vi "bats.parser.test.vi"() -> ()   [LabVIEW 2020]
uses:
  <vilib>/Platform/TimedLoop/XDataNode/XDataNode.xnode
  <vilib>/Platform/TimedLoop/XDataNode/nitl_modes.ctl
  <vilib>/Platform/TimedLoop/XDataNode/XDNodeRunTimeDep.lvlib
  <vilib>/Platform/TimedLoop/XDataNode/wakeup.ctl
  <vilib>/Platform/TimedLoop/XDataNode/timing_clust.ctl
  <vilib>/rvi/LocalResourceManager/LocalResourceManager.xnode
  <vilib>/rvi/DataTransferAndStorage/Container/XNode/niFpgaContainer.xnode
  <vilib>/rvi/FIFO/Fifo_Resource/niFpgaFifoEmulationRefIn.vi
  <vilib>/rvi/interface/RandomDataEmulation/nirviRandomDataFpgaMultiElementTemplate.vi
  <vilib>/rvi/FIFO/Fifo_Resource/nirvififoEmulationRead.vi
  Market.Data.Common/fpga/fpganow.common.fpga.lvlib
  <instrlib>/_niInstr/Network/IPv4/UDP/Data Stream/v1/niInstr IPv4 UDP Data Stream v1.lvclass
  <instrlib>/_niInstr/Network/IPv4/UDP/Data Stream/v1/Write Data Stream.vi
  <vilib>/rvi/DataTransferAndStorage/Container/Common/niFpgaContainerGetUniqueNameForEmu.vi
  <vilib>/rvi/DataTransferAndStorage/Container/Common/niFpgaContainerSetEmuInfo.vi
  <vilib>/rvi/eio/common/nirviEmuReportErrorAndStop.vi
  <instrlib>/_niInstr/Network/Ethernet/Utility/v1/FPGA/Network Data Stream.ctl
  <instrlib>/_niInstr/Network/Ethernet/Utility/v1/FPGA/niInstr Ethernet Utilities FPGA v1.lvlib
panel:
  out "byte":u8[](array[numeric]) format="%.0x"
  out "enabled":bool[](array[boolean])
  in  "Data Stream":T1={"data"=[0, 0, 0, 0, 0, 0, 0, 0], "data valid"=FALSE, "byte enables"=[FALSE, FALSE, FALSE, FALSE, FALSE, FALSE, FALSE, FALSE]}
  in  "niInstr IPv4 UDP Data Stream out":refnum<class "niInstr IPv4 UDP Data Stream v1.lvclass">
  out "Element":u64[](array[numeric])
  in  "reset":bool
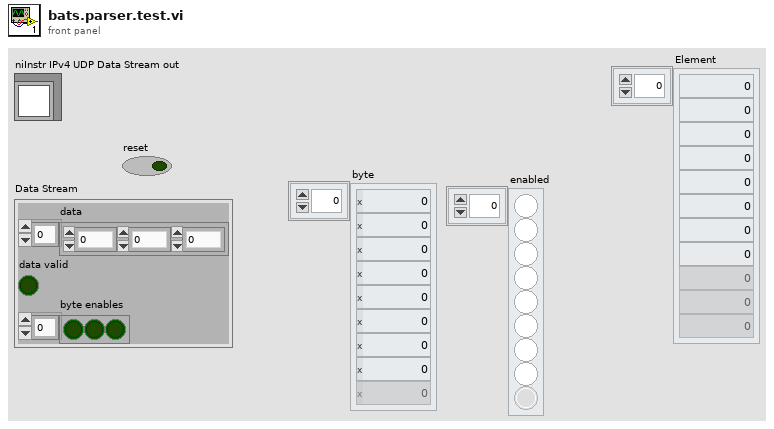
[diagram p1: front panel]
types:
  T1 = typedef "niInstr Ethernet Utilities FPGA v1.lvlib/Network Data Stream.ctl" = cluster{"data":u8[], "data valid":bool, "byte enables":bool[]}
  T2 = typedef "XDNodeRunTimeDep.lvlib/timing_clust.ctl" = cluster{"Expected End [f-1]":u64, "Actual End [f-1]":u64, "Finished Late? [f-1]":bool, "Expected End [i-1]":u64, "Actual End [i-1]":u64, "Finished Late? [i-1]":bool, "Expected Start [i]":u64, "Actual Start [i]":u64, "Expected Start [f]":u64, "Actual Start [f]":u64, "Source Name":string, "Structure Name":string, "Period":i64, "Deadline":i64, "Offset":i64, "Start":i64, "Priority":i32, "Timeout":i32, "Mode":T3, "Wakeup Reason":T4, "Error":errorcluster, "Source Type":string, "Secondary Source Type":string, "Global End Time":u64, "Global Start Time":u64, "Frame Duration":u64, "Iteration Duration":u64, "Assigned CPU":i32, "I/O Scan Engine Mode":u32}
  T3 = typedef "XDNodeRunTimeDep.lvlib/nitl_modes.ctl" = enum32{"No Change", "Process missed periods, maintain original phase", "Discard missed periods, maintain original phase", "Process missed periods, ignore original phase", "Discard missed periods, ignore original phase"}
  T4 = typedef "XDNodeRunTimeDep.lvlib/wakeup.ctl" = enum32{"Normal", "Aborted", "Asynchronous wakeup", "Timing source error", "Timed loop error", "Timeout"}
  T5 = typedef "fpganow.common.fpga.lvlib/u64.data.ctl" = cluster{"enabled":bool[], "byte":u8[]}
  T6 = cluster{"type":enum8{"Time", "AddOrder", "OrderExecuted", "OrderExecutedAtPrice", "ReduceSize", "ModifyOrder", "DeleteOrder", "Get.Everything", "Get.All.Orders", "Get.Top"}, "side":u8, "orderId ":u64, "quantity":u32, "symbol":u64, "price":u64, "executed.qty":u32, "canceled.qty":u32, "remaining.qty":u32, "seconds":u64, "nanoseconds":u64, "Add":bool, "Edit":bool, "Remove":bool, "seq no":u32}
  T7 = enum8{"Time", "AddOrder", "OrderExecuted", "OrderExecutedAtPrice", "ReduceSize", "ModifyOrder", "DeleteOrder", "Get.Everything", "Get.All.Orders", "Get.Top"}
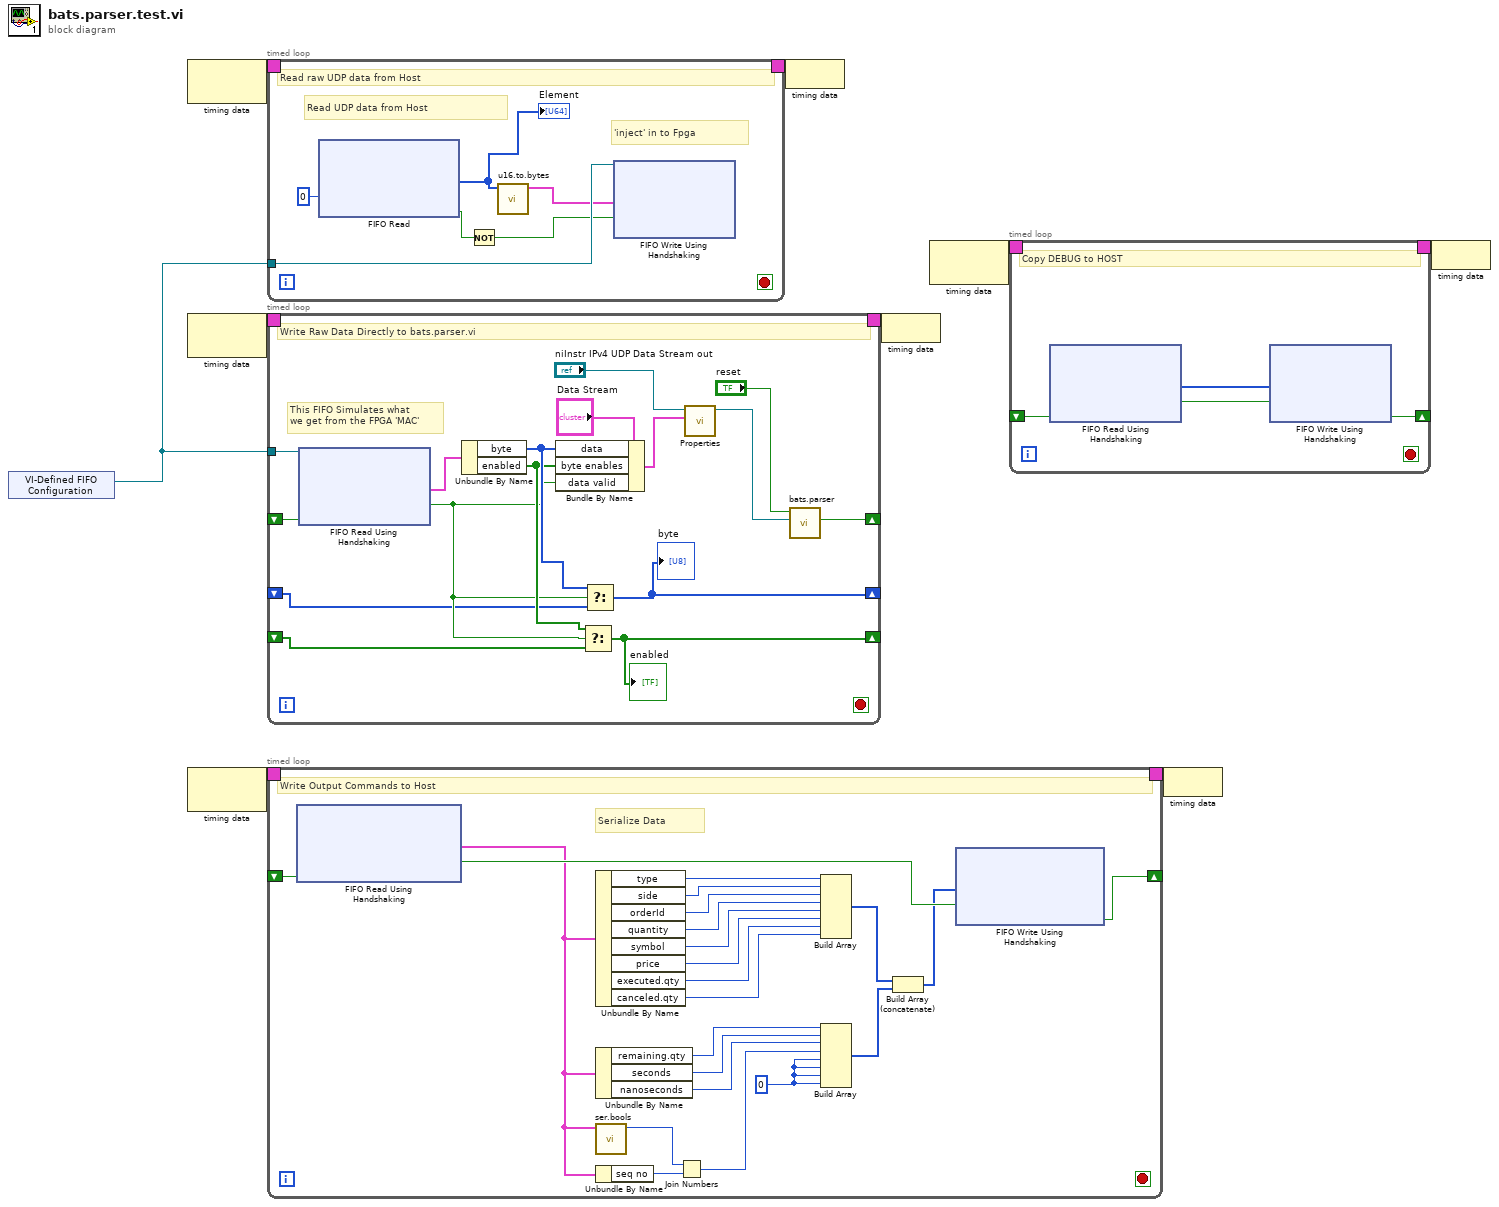
[diagram p0: block diagram]
diagram:
  n1 = xnode "VI-Defined FIFO Configuration"() -> ("FIFO Out"=w5:refnum<k21>)
  n2 = node-c288() -> (w9:T2)  [unwired: 1 in]
  n3 = node-c288() -> (w7:T2)  [unwired: 1 in]
  n4 = node-c288() -> (w4:T2)  [unwired: 1 in]
  n5 = timed-loop {
    timing: w9 -> [_]
    timing-out: [_] -> w8
    tunnel: w5 -> [w15]
    stop <- _ stop-if-true
    # "'inject' in to Fpga"
    # "Read UDP data from Host"
    # "Read raw UDP data from Host"
    n6 = xnode ("FIFO Read")("Timeout"=0) -> ("Element"=w11:u64[], "Timed Out?"=w13:bool)  [unwired: 1 in, 1 out]
    "Element" <- w11
    n7 = Not(x=w13) -> (.not. x?=w12:bool)
    n8 = call "u16.to.bytes.vi"("data.u16.in"=w11) -> ("data"=w10:T5)  [unwired: 10 in]
    n9 = xnode ("FIFO Write Using Handshaking")("Element"=w10, "Input Valid"=w12, "FIFO In"=w15) -> ()  [unwired: 2 out]
  }
  n10 = timed-loop {
    timing: w7 -> [_]
    timing-out: [_] -> w6
    tunnel: w5 -> [w33]
    shift-right: [w32] -> _
    shift-left: _ -> [w29]
    shift-right: [w21] -> _
    shift-left: _ -> [w19]
    shift-right: [w20] -> _
    shift-left: _ -> [w18]
    stop <- _ stop-if-true
    # "This FIFO Simulates what\nwe get from the FPGA 'MAC'"
    # "Write Raw Data Directly to bats.parser.vi"
    n11 = xnode ("FIFO Read Using Handshaking")("Ready for Output"=w29, "FIFO In"=w33) -> ("Element"=w30:cluster{"enabled":bool[], "byte":u8[]}, "Output Valid"=w22:bool)  [unwired: 1 out]
    n12 = Unbundle By Name(w30) -> ("byte"=w24:u8[], "enabled"=w23:bool[])
    n13 = Bundle By Name(cluster="Data Stream", "data"=w24, "byte enables"=w23, "data valid"=w22) -> (w28:T1)
    n14 = Select(t=w23, s=w22, f=w18) -> (s? t:f=w20:bool[])
    "enabled" <- w20
    n15 = Select(t=w24, s=w22, f=w19) -> (s? t:f=w21:u8[])
    "byte" <- w21
    n16 = call-poly <instrlib>:"Properties.vi"("Data Stream"=w28, "niInstr IPv4 Data Stream in"="niInstr IPv4 UDP Data Stream out") -> ("niInstr IPv4 Data Stream out"=w25:refnum<class "niInstr IPv4 UDP Data Stream v1.lvclass">)  [unwired: 9 in]
    n17 = call "bats.parser.vi"("data.stream"=w25, "reset"="reset") -> ("Ready.for.Udp.Input"=w32:bool)  [unwired: 9 in]
  }
  n18 = timed-loop {
    timing: w4 -> [_]
    timing-out: [_] -> w3
    shift-right: [w57] -> _
    shift-left: _ -> [w48]
    stop <- _ stop-if-true
    w42 = u64 0 ("element")
    # "Serialize Data"
    # "Write Output Commands to Host"
    n19 = xnode ("FIFO Read Using Handshaking")("Ready for Output"=w48) -> ("Element"=w37:T6, "Output Valid"=w47:bool)  [unwired: 1 in, 1 out]
    n20 = Unbundle By Name(w37) -> ("type"=w56:T7, "side"=w55:u8, "orderId"=w54:u64, "quantity"=w53:u32, "symbol"=w52:u64, "price"=w51:u64, "executed.qty"=w50:u32, "canceled.qty"=w49:u32)
    n21 = Unbundle By Name(w37) -> ("remaining.qty"=w43:u32, "seconds"=w40:u64, "nanoseconds"=w41:u64)
    n22 = call "ser.bools.vi"("orderbook.command"=w37) -> ("Numeric"=w38:u32)  [unwired: 10 in]
    n23 = Unbundle By Name(w37) -> ("seq no"=w36:u32)
    n24 = Join Numbers(hi=w38, lo=w36) -> ((hi.lo)=w39:u64)
    n25 = Build Array(w56, w55, w54, w53, w52, w51, w50, w49) -> (w46:u64[])
    n26 = Build Array(w43, w40, w41, w39, w42, w42, w42, w42) -> (w44:u64[])
    n27 = Build Array (concatenate)(w46, w44) -> (w45:u64[])
    n28 = xnode ("FIFO Write Using Handshaking")("Element"=w45, "Input Valid"=w47) -> ("Ready for Input"=w57:bool)  [unwired: 1 in, 1 out]
  }
  n29 = node-c288(w8) -> ()
  n30 = node-c288(w6) -> ()
  n31 = node-c288() -> (w2:T2)  [unwired: 1 in]
  n32 = timed-loop {
    timing: w2 -> [_]
    timing-out: [_] -> w1
    shift-right: [w63] -> _
    shift-left: _ -> [w62]
    stop <- _ stop-if-true
    # "Copy DEBUG to HOST"
    n33 = xnode ("FIFO Read Using Handshaking")("Ready for Output"=w62) -> ("Element"=w60:u64[], "Output Valid"=w61:bool)  [unwired: 1 in, 1 out]
    n34 = xnode ("FIFO Write Using Handshaking")("Element"=w60, "Input Valid"=w61) -> ("Ready for Input"=w63:bool)  [unwired: 1 in, 1 out]
  }
  n35 = node-c288(w3) -> ()
  n36 = node-c288(w1) -> ()
